vi "FOCUS_V42_H37.vi"(9 "X-pixels":sgl=256.0, 11 "Run":bool) -> (0 "Retrace pixels":sgl, 10 "Pixel Clock (Hz)":sgl)   [LabVIEW 2010] (continued)
            n1001 = Array Max & Min(array=w3025) -> (max value=w3029:dbl, min value=w3028:dbl)  [unwired: 2 out]
            n1002 = Greater?(x=w3029, y=w3022) -> (0:w3027:bool)
            n1003 = Less?(x=w3028, y=w3023) -> (x < y?=w3026:bool)
            n1004 = Or(x=w3027, y=w3026) -> (x .or. y?=w3024:bool)
            n1005 = case shown="False" w3024 {
              tunnel: [u32 16711680 u32 0] -> w3030
              frame True {
              }
              frame False {
                (unwired) u32 16756736
              }
            }
          }
        }
        n1006 = Bundle(w2040, w2041) -> (→"Galvos":cluster{dbl[], dbl[]})  [unwired: 1 in]
        n1007 = local read "frame/line indicator"() -> (w2025:u16)
        n1008 = local read "frame/line indicator"() -> (w1885:u16)
        n1009 = property class="DAQmx Buffer"(reference=w1952, error in=w1950, "Input:Buffer Size"=u32 10000000 ("Input.BufSize")) -> (reference out=w1951:refnum<k21>, error out=w1949:errorcluster)
        n1010 = Concatenate Strings(w1897, tag "/PXI_Trig2" ("source terminal")) -> (w1989:string)
        n1011 = call-poly <vilib>:"DAQmx Create Channel (CO-Pulse Generation-Ticks).vi"("high ticks"=w1877, "low ticks"=w1875, "counter"=w1935, "source of ticks"=w1929, "error in"=w1924, "initial delay"=w1878) -> ("task out"=w1961:refnum<k21>, "error out"=w1960:errorcluster)  [unwired: 8 in]
        n1012 = Greater Or Equal?(x=w2025, y=3.0) -> (x >= y?=w2024:bool)
        n1013 = Concatenate Strings(w1897, tag "/PXI_Trig2" ("destination terminal")) -> (w1993:string)
        n1014 = Bundle("Trigger?"="Trigger?", "Type"="Type", "Level [V]"="Level [V]", "slope"="slope") -> (w1908:T17)  [unwired: 1 in]
        n1015 = Type Cast(type=tag "" ("destination terminal"), x=w1989) -> (*(type *) &x=w1986:tag)
        n1016 = Concatenate Strings(w1897, tag "/10MHzRefClock" ("source terminal")) -> (w1998:string)
        n1017 = Type Cast(type=tag "" ("destination terminal"), x=w1993) -> (*(type *) &x=w1990:tag)
        n1018 = Type Cast(type=tag "" ("destination terminal"), x=w1998) -> (*(type *) &x=w1995:tag)
        n1019 = call-poly <vilib>:"DAQmx Timing (Implicit).vi"("task/channels in"=w1961, "sample mode"=w1959, "error in"=w1960) -> ("task out"=w1958:refnum<k21>, "error out"=w1957:errorcluster)  [unwired: 11 in]
        n1020 = case shown="3" w1885 {
          tunnel: [_ _ w3015 w3018 w3019] -> w2030
          frame 0, Default {
          }
          frame 1 {
          }
          frame 2 {
            n1021 = local read "Y-lines"() -> (w3016:sgl)
            n1022 = local read "Number of frames"() -> (w3017:sgl)
            n1023 = Multiply(x=w3016, y=w3017) -> (x*y=w3015:sgl)
          }
          frame 3 {
            n1024 = local read "Y-lines FreeLine"() -> (w3018:sgl)
          }
          frame 4 {
            n1025 = local read "Y-lines FreeLine"() -> (w3019:sgl)
          }
        }
        n1026 = local read "Fiberscope\nMode"() -> (w1894:bool)
        n1027 = case shown="False" w1894 {
          tunnel: w2024 -> [w2081 _]
          tunnel: w1947 -> [w2080 _]
          tunnel: [w2079 w2084] -> w1916
          frame False {
            n1028 = case shown="False" w2081 {
              tunnel: [w2082 w2083] -> w2079
              tunnel: w2080 -> [_ _]
              frame False {
                n1029 = local read "Pixel Clock (Hz)"() -> (w2082:sgl)
              }
              frame True {
                n1030 = local read "Pixel Clock (Hz) FreeLine"() -> (w2083:sgl)
              }
            }
          }
          frame True {
            n1031 = local read "Pixel Clock (Hz) FScope"() -> (w2084:sgl)
          }
        }
        n1032 = case shown="True" w1917 {
          tunnel: [_ w2978] -> w2014
          tunnel: [_ w2977] -> w2013
          tunnel: w1916 -> [_ w2974]
          tunnel: w1922 -> [_ w2962]
          frame False {
          }
          frame True {
            w2981 = 10123 items=["Finite Samples"=10178, "Continuous Samples"=10123, "Hardware Timed Single Point"=12522] ("sample mode")
            w2982 = 10171 items=["Rising"=10280, "Falling"=10171] ("edge")
            n1033 = local read "AI Device"() -> (w2949:tag)
            n1034 = Concatenate Strings(w2949, tag "/ai0," ("physical channels"), w2949, tag "/ai1," ("physical channels"), w2949, tag "/ai2," ("physical channels"), w2949, tag "/ai3" ("physical channels")) -> (w2971:string)
            n1035 = Type Cast(type=tag "" ("physical channels"), x=w2971) -> (*(type *) &x=w2968:tag)
            n1036 = local read "AO/DIO Device"() -> (w2952:tag)
            n1037 = call-poly <vilib>:"DAQmx Create Channel (AI-Voltage-Basic).vi"("maximum value"=10.0, "physical channels"=w2968, "error in"=w2962) -> ("task out"=w2979:refnum<k21>, "error out"=w2980:errorcluster)  [unwired: 11 in]
            n1038 = Concatenate Strings(tag "/" ("destination terminal"), w2952, tag "/ao/SampleClock" ("source")) -> (w2953:string)
            n1039 = Type Cast(type=tag "" ("source"), x=w2953) -> (*(type *) &x=w2951:tag)
            n1040 = call-poly <vilib>:"DAQmx Timing (Sample Clock).vi"("task/channels in"=w2979, "sample mode"=w2981, "rate"=w2974, "source"=w2951, "error in"=w2980) -> ("task out"=w2961:refnum<k21>, "error out"=w2960:errorcluster)  [unwired: 9 in]
            n1041 = property class="DAQmx Buffer"(reference=w2961, error in=w2960, "Input:Buffer Size"=u32 5000000 ("Input.BufSize")) -> (reference out=w2958:refnum<k21>, error out=w2959:errorcluster)
            n1042 = Concatenate Strings(tag "/" ("destination terminal"), w2952, tag "/ao/StartTrigger" ("source")) -> (w2967:string)
            n1043 = Type Cast(type=tag "" ("source"), x=w2967) -> (*(type *) &x=w2965:tag)
            n1044 = call-poly <vilib>:"DAQmx Start Trigger (Digital Edge).vi"("task/channels in"=w2958, "source"=w2965, "edge"=w2982, "error in"=w2959) -> ("task out"=w2976:refnum<k21>, "error out"=w2975:errorcluster)  [unwired: 10 in]
            n1045 = call <vilib>:"DAQmx Start Task.vi"("task/channels in"=w2976, "error in"=w2975) -> ("task out"=w2978:refnum<k21>, "error out"=w2977:errorcluster)  [unwired: 12 in]
          }
        }
        n1046 = call "AOConfigwriteDAQmx.vi"("AO.UseOnlyOnBrdMem"=FALSE, "TriggerCluster"=w1908, "Trigger Source"=w1907, "Sampling"=w1915, "rate"=w1916, "data"=w1889, "error in"=w1922, "RegenMode"=w2027, "Output.OnbrdBufSize"=w1947, "physical channels"=w2015) -> ("error out"=w2009:errorcluster, "task out"=w2008:refnum<k21>)
        n1047 = call <vilib>:"DAQmx Connect Terminals.vi"("source terminal"=w1995, "destination terminal"=w1990, "error in"=w2009) -> ("error out"=w2028:errorcluster)  [unwired: 12 in]
        n1048 = Concatenate Strings(w1897, tag "/ao/StartTrigger" ("source terminal")) -> (w1900:string)
        n1049 = call <vilib>:"DAQmx Start Task.vi"("task/channels in"=w1958, "error in"=w1957) -> ("task out"=w1956:refnum<k21>, "error out"=w1923:errorcluster)  [unwired: 12 in]
        n1050 = call-poly <vilib>:"DAQmx Timing (Sample Clock).vi"("task/channels in"=w1951, "sample mode"=w2012, "rate"=w1916, "source"=w1964, "error in"=w1949) -> ("task out"=w2011:refnum<k21>, "error out"=w2010:errorcluster)  [unwired: 9 in]
        n1051 = Concatenate Strings(w1897, tag "/PFI2" ("destination terminal")) -> (w1985:string)
        n1052 = Type Cast(type=tag "" ("destination terminal"), x=w1900) -> (*(type *) &x=w1896:tag)
        n1053 = Concatenate Strings(w1897, tag "/PFI5" ("destination terminal")) -> (w1977:string)
        n1054 = Concatenate Strings(w1897, tag "/PFI7" ("destination terminal")) -> (w1906:string)
        n1055 = local read "frame/line indicator"() -> (w2038:u16)
        n1056 = Type Cast(type=tag "" ("destination terminal"), x=w1985) -> (*(type *) &x=w1982:tag)
        n1057 = call <vilib>:"DAQmx Connect Terminals.vi"("source terminal"=w1986, "destination terminal"=w1982, "error in"=w2028) -> ("error out"=w1903:errorcluster)  [unwired: 12 in]
        n1058 = property on="Galvos" class="XYGraph (strict)"("Plot Area:Colors:FG Color"=w2042, "Plot Area:Colors:BG Color"=w2042) -> ()  [unwired: 2 in, 2 out]
        n1059 = Concatenate Strings(w1897, tag "/ao/SampleClock" ("source terminal")) -> (w1981:string)
        n1060 = Type Cast(type=tag "" ("destination terminal"), x=w1977) -> (*(type *) &x=w1974:tag)
        n1061 = Type Cast(type=tag "" ("destination terminal"), x=w1906) -> (*(type *) &x=w1901:tag)
        n1062 = call <vilib>:"DAQmx Connect Terminals.vi"("source terminal"=w1896, "destination terminal"=w1901, "error in"=w1903) -> ("error out"=w1902:errorcluster)  [unwired: 12 in]
        n1063 = call <vilib>:"DAQmx Start Task.vi"("task/channels in"=w2011, "error in"=w2010) -> ("task out"=w2017:refnum<k21>, "error out"=w2016:errorcluster)  [unwired: 12 in]
        n1064 = for {
          N: w2030 -> [_]
          tunnel: [w3020] -> w2031 mode=indexing
          i -> [w3020]
        }
        n1065 = Type Cast(type=tag "" ("destination terminal"), x=w1981) -> (*(type *) &x=w1978:tag)
        n1066 = call <vilib>:"DAQmx Connect Terminals.vi"("source terminal"=w1978, "destination terminal"=w1974, "error in"=w1902) -> ()  [unwired: 12 in, 1 out]
      }
    }
    n1067 = local read "Image3Array"() -> (w171:u8[][])
    n1068 = local read "Image4Array"() -> (w187:u8[][])
    n1069 = local read "Image1Array"() -> (w176:u8[][])
    n1070 = local read "Image2Array"() -> (w186:u8[][])
    n1071 = flat-sequence {
      tunnel: w176 -> [_]
      frame #0 {
        n1072 = property on="Property Node" class="VI"() -> ("VI Path"=w330:path)  [unwired: 2 in, 2 out]
        n1073 = Initialize Array(u8 0 ("x 2")) -> (w315:u8[])  [unwired: 1 in]
        n1074 = Strip Path(path=w330) -> (stripped path=w306:path)  [unwired: 1 out]
        n1075 = local read "VISA Sutter MP-285"() -> (w321:refnum<visa-resource-name>)
        n1076 = local read "MaiTai setting Path"() -> (w317:path)
        n1077 = local read "VISA XPG-ADC"() -> (w319:refnum<visa-resource-name>)
        n1078 = Strip Path(path=w306) -> ()  [unwired: 2 out]
        n1079 = local read "AO/DIO Device"() -> (w334:tag)
        n1080 = local read "AI Device"() -> (w327:tag)
        n1081 = Build Path(base path=w306, name or relative path="FOCUS.cfg") -> (appended path=w310:path)
        n1082 = Path To String(path=w317) -> (string=w316:string)
        n1083 = Type Cast(type="" ("name or relative path"), x=w319) -> (*(type *) &x=w318:string)
        n1084 = Type Cast(type="" ("name or relative path"), x=w321) -> (*(type *) &x=w320:string)
        n1085 = Type Cast(type=w315, x=w327) -> (*(type *) &x=w301:u8[])
        n1086 = Type Cast(type=w315, x=w316) -> (*(type *) &x=w314:u8[])
        n1087 = Type Cast(type=w315, x=w318) -> (*(type *) &x=w324:u8[])
        n1088 = Type Cast(type=w315, x=w320) -> (*(type *) &x=w325:u8[])
        n1089 = Type Cast(type=w315, x=w334) -> (*(type *) &x=w305:u8[])
        n1090 = Array Size(array=w301) -> (size(s)=w302:i32)
        n1091 = Array Size(array=w314) -> (size(s)=w313:i32)
        n1092 = Array Size(array=w305) -> (size(s)=w304:i32)
        n1093 = To Unsigned Byte Integer(number=w302) -> (unsigned 8bit integer=w300:u8)
        n1094 = To Unsigned Byte Integer(number=w313) -> (unsigned 8bit integer=w312:u8)
        n1095 = call <vilib>:"Open_Create_Replace File.vi"("advisory dialog? (display:T)"=FALSE, "function (open:0)"=T8."create or replace", "file path"=w310) -> ("error out"=w308:errorcluster, "refnum"=w309:refnum<file>)  [unwired: 5 in, 2 out]
        n1096 = To Unsigned Byte Integer(number=w304) -> (unsigned 8bit integer=w303:u8)
        n1097 = Build Array (concatenate)(w303, w305, w300, w301, w325, w324, w312, w314) -> (w326:u8[])
        n1098 = Write to Binary File(file (use dialog)=w309, data=w326, error in=w308, 5:FALSE ("prepend array or string size? (T)")) -> (refnum out=w328:refnum<file>, error out=w329:errorcluster)  [unwired: 2 in, 1 out]
        n1099 = Close File(refnum=w328, error in=w329) -> (error out=w332:errorcluster)  [unwired: 1 out]
        n1100 = call <vilib>:"Simple Error Handler.vi"("error in (no error)"=w332) -> ()  [unwired: 4 in, 5 out]
      }
    }
    n1101 = Equal?(x=w182, y=u16 4) -> (x = y?=w180:bool)
    n1102 = local read "ScanLineFreeLine"() -> (w198:sgl[][])
    n1103 = Index Array(array=w198, index (row)=0 ("disabled index (col)")) -> (element=w197:sgl[])  [unwired: 1 in]
    n1104 = Index Array(array=w198, index (row)=1 ("disabled index (col)")) -> (element=w178:sgl[])  [unwired: 1 in]
    n1105 = case shown="False" w180 {
      tunnel: [w335 w339] -> w179
      tunnel: w178 -> [w336 _]
      frame False {
        n1106 = Array Size(array=w336) -> (size(s)=w337:i32)
        n1107 = Initialize Array(sgl 0.0 ("element"), w337) -> (w335:sgl[])
      }
      frame True {
        n1108 = local read "Zsin3D"() -> (w339:sgl[])
      }
    }
    n1109 = Greater Or Equal?(x=w182, y=u16 3) -> (x >= y?=w183:bool)
    n1110 = local write "Ready?"(FALSE ("Ready?")) -> ()
    n1111 = property on="Image 2" class="IntGraph (strict)"() -> ("Color Table"=w289:u32[])  [unwired: 2 in, 2 out]
    n1112 = Interleave 1D Arrays(w197, w178, w179) -> (w193:sgl[])
    n1113 = local read "Positions"() -> (w192:sgl[])
    n1114 = local read "Focus"() -> (w208:bool)
    n1115 = local write "OpenShutter"(FALSE ("OpenShutter")) -> ()
    n1116 = local read "Channel selector"() -> (w160:u8)
    n1117 = Array Size(array=w193) -> (size(s)=w194:i32)
    n1118 = local write "Run"(w208) -> ()
    n1119 = Build Array (concatenate)(w194, w193, w192) -> (w185:sgl[])
    n1120 = flat-sequence {
      tunnel: [w431] -> w296
      tunnel: [w430] -> w163
      tunnel: [w398] -> w292
      tunnel: [w399] -> w291
      tunnel: w289 -> [w409]
      tunnel: w259 -> [w426]
      tunnel: w288 -> [w425]
      tunnel: [w424] -> w287
      tunnel: [w423] -> w286
      tunnel: w283 -> [w422]
      tunnel: w282 -> [w421]
      tunnel: [w400] -> w277
      tunnel: [w401] -> w276
      tunnel: [w387] -> w264
      tunnel: [w404] -> w219
      tunnel: [w403] -> w218
      tunnel: [w402] -> w210
      tunnel: w207 -> [w381]
      tunnel: w171 -> [w380]
      tunnel: w187 -> [w379]
      tunnel: w176 -> [w378]
      tunnel: w186 -> [w377]
      tunnel: w185 -> [w376]
      tunnel: w183 -> [w375]
      tunnel: w168 -> [w363]
      tunnel: [w363] -> w167
      tunnel: [w357] -> w161
      tunnel: w160 -> [w356]
      frame #0 {
        w408 = FALSE ("data")
        w420 = i8 -1 ("element")
        n1121 = local read "Mode selector"() -> (w372:u16)
        n1122 = local read "frame/line indicator"() -> (w428:u16)
        n1123 = local read "ImageSelector"() -> (w417:bool)
        n1124 = Split Number(x=w409) -> (lo(x)=w411:u16[])  [unwired: 1 out]
        n1125 = Split Number(x=w411) -> (lo(x)=w410:u8[])  [unwired: 1 out]
        n1126 = Equal?(x=w428, y=4) -> (x = y?=w362:bool)
        n1127 = Equal?(x=w372, y=4) -> (x = y?=w359:bool)
        n1128 = Or(x=w362, y=w363) -> (x .or. y?=w361:bool)
        n1129 = property on="Intensity" class="Slide (strict)"("Scale.Range:Maximum"="IntensityScaleMax") -> ()  [unwired: 2 in, 2 out]
        n1130 = Not(x=w359) -> (.not. x?=w360:bool)
        n1131 = And(x=w360, y=w361) -> (x .and. y?=w358:bool)
        n1132 = case shown="False" w358 {
          tunnel: [w456 _] -> w396
          tunnel: [w455 _] -> w397
          tunnel: w359 -> [w454 _]
          frame False {
            n1133 = case shown="True" w454 {
              tunnel: [w466 w479] -> w456
              tunnel: [w465 w478] -> w455
              frame False {
                n1134 = local read "AO/DIO Device"() -> (w462:tag)
                n1135 = Concatenate Strings(w462, tag "/ao3" ("physical channels")) -> (w460:string)
                n1136 = Type Cast(type=tag "" ("physical channels"), x=w460) -> (*(type *) &x=w458:tag)
                n1137 = call-poly <vilib>:"DAQmx Create Channel (AO-Voltage-Basic).vi"("physical channels"=w458) -> ("task out"=w463:refnum<k21>, "error out"=w464:errorcluster)  [unwired: 13 in]
                n1138 = local read "Intensity"() -> (w457:sgl)
                n1139 = call-poly <vilib>:"DAQmx Write (Analog DBL 1Chan 1Samp).vi"("task/channels in"=w463, "data"=w457, "error in"=w464) -> ("task out"=w466:refnum<k21>, "error out"=w465:errorcluster)  [unwired: 10 in, 1 out]
              }
              frame True {
                n1140 = local read "AO/DIO Device"() -> (w467:tag)
                n1141 = Concatenate Strings(w467, tag "/ao2," ("physical channels"), w467, tag "/ao3" ("physical channels")) -> (w474:string)
                n1142 = Type Cast(type=tag "" ("physical channels"), x=w474) -> (*(type *) &x=w472:tag)
                n1143 = call-poly <vilib>:"DAQmx Create Channel (AO-Voltage-Basic).vi"("physical channels"=w472) -> ("task out"=w476:refnum<k21>, "error out"=w477:errorcluster)  [unwired: 13 in]
                n1144 = local read "Intensity"() -> (w470:sgl)
                n1145 = Build Array(sgl 0.0 ("element"), w470) -> (w469:sgl[])
                n1146 = call-poly <vilib>:"DAQmx Write (Analog 1D DBL NChan 1Samp).vi"("task/channels in"=w476, "data"=w469, "error in"=w477) -> ("task out"=w479:refnum<k21>, "error out"=w478:errorcluster)  [unwired: 10 in, 1 out]
              }
            }
          }
          frame True {
          }
        }
        n1147 = local read "Fiberscope\nMode"() -> (w402:bool)
        n1148 = call "VISA MP-285 GetSet Speed.vi"("Input: Duty Cluster"=w381, "Input: Speed in microns/sec"="Sutter Speed [um/s]") -> ("Output: Duty Cluster"=w391:T18)  [unwired: 1 out]
        n1149 = call "VISA MP-285 Get Position.vi"("Input: Duty Cluster"=w391) -> ("Output: X axis (microns)"=w383:dbl, "Output: Y axis (microns)"=w384:dbl, "Output: Z axis (microns)"=w389:dbl, "Output: Duty Cluster"=w388:T18)
        n1150 = Multiply(x=w383, y="Sutter scale x") -> (x*y=→"x-positionstart (um)":dbl)
        n1151 = Multiply(x=w384, y="Sutter scale y") -> (x*y=→"y-positionstart (um)":dbl)
        n1152 = local read "frame scan finished?"() -> (w371:bool)
        n1153 = Multiply(x="Sutter scale z", y=w389) -> (x*y=w382:dbl)
        "z-positionstart (um)" <- w382
        n1154 = local read "AO/DIO Device"() -> (w414:tag)
        n1155 = property on="ImageSlide" class="Slide (strict)"() -> ("Scale.Range:Maximum"=w419:dbl, "Visible"=w418:bool)  [unwired: 2 in, 2 out]
        n1156 = case shown="True" w402 {
          tunnel: [_ w448] -> w404
          tunnel: [_ w447] -> w403
          frame False {
          }
          frame True {
            w442 = TRUE ("element")
            n1157 = local read "AO/DIO Device"() -> (w444:tag)
            n1158 = Concatenate Strings(w444, tag "/port2/line6," ("lines"), w444, tag "/port2/line7" ("lines")) -> (w453:string)
            n1159 = Type Cast(type=tag "" ("lines"), x=w453) -> (*(type *) &x=w451:tag)
            n1160 = call-poly <vilib>:"DAQmx Create Channel (DO-Digital Output).vi"("lines"=w451) -> ("task out"=w450:refnum<k21>, "error out"=w449:errorcluster)  [unwired: 13 in]
            n1161 = Build Array(w442, w442) -> (w443:bool[])
            n1162 = call-poly <vilib>:"DAQmx Write (Digital 1D Bool 1Chan 1Samp).vi"("task/channels in"=w450, "data"=w443, "error in"=w449) -> ("task out"=w448:refnum<k21>, "error out"=w447:errorcluster)  [unwired: 10 in, 1 out]
          }
        }
        n1163 = Concatenate Strings(w414, tag "/port1/line1" ("lines")) -> (w416:string)
        n1164 = local read "GetFirst"() -> (w385:bool)
        n1165 = local read "GetLast"() -> (w386:bool)
        n1166 = Type Cast(type=tag "" ("lines"), x=w416) -> (*(type *) &x=w412:tag)
        n1167 = And(x=w371, y="Go back?") -> (x .and. y?=w369:bool)
        n1168 = And(x=w385, y=w386) -> (x .and. y?=w374:bool)
        n1169 = call-poly <vilib>:"DAQmx Create Channel (DO-Digital Output).vi"("lines"=w412) -> ("task out"=w407:refnum<k21>, "error out"=w406:errorcluster)  [unwired: 13 in]
        "Shutter" <- w407
        n1170 = Or(x=w369, y=w374) -> (x .or. y?=w367:bool)
        n1171 = case shown="True" w367 {
          tunnel: w388 -> [w433 w441]
          tunnel: [w433 w440] -> w387
          tunnel: w382 -> [_ w438]
          tunnel: [FALSE ("IntDevUsed 2") FALSE ("IntDevUsed 2")] -> w368
          frame False {
          }
          frame True {
            n1172 = local read "FirstPosition"() -> (w437:sgl)
            n1173 = local read "Sutter scale z"() -> (w434:sgl)
            n1174 = Subtract(x=w437, y=w438) -> (x-y=w436:dbl)
            n1175 = Divide(x=w436, y=w434) -> (x/y=w439:dbl)
            n1176 = call "VISA MP-285 Step.vi"("Input: Duty Cluster"=w441, "Input: Delta Z axis (microns)"=w439) -> ("Output: Duty Cluster"=w440:T18)  [unwired: 2 in, 3 out]
          }
        }
        n1177 = local write "frame scan finished?"(w368) -> ()
        n1178 = local write "Shutter open"(w408) -> ()
        n1179 = call-poly <vilib>:"DAQmx Write (Digital Bool 1Line 1Point).vi"("task/channels in"=w407, "data"=w408, "error in"=w406) -> ("task out"=w394:refnum<k21>, "error out"=w395:errorcluster)  [unwired: 10 in, 1 out]
        n1180 = while {
          tunnel: ["Run"] -> w431
          tunnel: ["End experiment"] -> w430
          shift-right: [w581] -> _
          shift-left: w409 -> [w584]
          shift-right: [w579] -> _
          shift-left: FALSE ("Visible") -> [w580]
          tunnel: w426 -> [w578]
          tunnel: w425 -> [w577]
          tunnel: [w578] -> w424
          tunnel: [w577] -> w423
          tunnel: w422 -> [w575]
          tunnel: w421 -> [w567]
          shift-right: [w540] -> _
          shift-left: w420 -> [w541]
          shift-right: [w538] -> _
          shift-left: w420 -> [w539]
          tunnel: w419 -> [w537]
          tunnel: w418 -> [w536]
          shift-right: [w529] -> _
          shift-left: w417 -> [w528]
          shift-right: [w522] -> _
          shift-left: w410 -> [w523]
          tunnel: [w502] -> w401
          tunnel: [w501] -> w400
          tunnel: [w506] -> w399
          tunnel: [w505] -> w398
          tunnel: w397 -> [w508]
          tunnel: w396 -> [w507]
          tunnel: w395 -> [w504]
          tunnel: w394 -> [w503]
          tunnel: w380 -> [w488]
          tunnel: w379 -> [w487]
          tunnel: w378 -> [w489]
          tunnel: w377 -> [w490]
          tunnel: w376 -> [w493]
          tunnel: w375 -> [w491]
          tunnel: [w481] -> w357
          shift-right: [w480] -> _
          shift-left: w356 -> [w482]
          i -> [w527]
          stop <- w518 stop-if-true
          n1181 = local read "index (row)1"() -> (w546:i32)
          n1182 = property on="Image 2" class="IntGraph (strict)"() -> ("Color Table"=w583:u32[])  [unwired: 2 in, 2 out]
          n1183 = event shown="[0] Timeout" {
            selector: _ -> [_ _ _ _ _ _ _ _ _ _ _ _ _ _ _ _ _ _ _ _ _ _ _ _ _ _ _ _ _ _ _ _ _ _ _]
            dyn-events: _ -> [_ _ _ _ _ _ _ _ _ _ _ _ _ _ _ _ _ _ _ _ _ _ _ _ _ _ _ _ _ _ _ _ _ _ _]
            timeout: 0 -> [_ _ _ _ _ _ _ _ _ _ _ _ _ _ _ _ _ _ _ _ _ _ _ _ _ _ _ _ _ _ _ _ _ _ _]
            tunnel: [FALSE ("Fiberscope\nMode") TRUE ("Fiberscope\nMode") TRUE ("Fiberscope\nMode") TRUE ("Fiberscope\nMode") TRUE ("Fiberscope\nMode") TRUE ("Fiberscope\nMode") TRUE ("Fiberscope\nMode") TRUE ("Fiberscope\nMode") TRUE ("Fiberscope\nMode") TRUE ("Fiberscope\nMode") TRUE ("Fiberscope\nMode") TRUE ("Fiberscope\nMode") TRUE ("Fiberscope\nMode") TRUE ("Fiberscope\nMode") TRUE ("Fiberscope\nMode") TRUE ("Fiberscope\nMode") TRUE ("Fiberscope\nMode") TRUE ("Fiberscope\nMode") TRUE ("Fiberscope\nMode") TRUE ("Fiberscope\nMode") TRUE ("Fiberscope\nMode") TRUE ("Fiberscope\nMode") TRUE ("Fiberscope\nMode") TRUE ("Fiberscope\nMode") TRUE ("Fiberscope\nMode") TRUE ("Fiberscope\nMode") TRUE ("Fiberscope\nMode") TRUE ("Fiberscope\nMode") TRUE ("Fiberscope\nMode") FALSE ("Fiberscope\nMode") _ FALSE ("Fiberscope\nMode") FALSE ("Fiberscope\nMode") FALSE ("Fiberscope\nMode") FALSE ("Fiberscope\nMode")] -> w510
            tunnel: [_ _ _ _ _ _ _ _ w657 _ _ _ _ _ _ _ _ _ _ _ _ _ _ _ _ _ _ _ _ _ _ _ _ _ _] -> w509
            tunnel: w508 -> [w615 w620 w625 w630 w635 w640 w645 w650 w655 w661 w666 w671 w676 w681 w686 w691 w696 w701 w706 w711 w716 w721 w726 w731 w736 w741 w746 w751 w757 w765 w770 w777 w797 w802 w809]
            tunnel: w507 -> [w616 w621 w626 w631 w636 w641 w646 w651 w656 w662 w667 w672 w677 w682 w687 w692 w697 w702 w707 w712 w717 w722 w727 w732 w737 w742 w747 w752 w758 w764 w771 w778 w798 w803 w810]
            tunnel: [w615 w620 w625 w630 w635 w640 w645 w650 w655 w661 w666 w671 w676 w681 w686 w691 w696 w701 w706 w711 w716 w721 w726 w731 w736 w741 w746 w751 w757 w763 w770 w777 w797 w802 w809] -> w506
            tunnel: [w616 w621 w626 w631 w636 w641 w646 w651 w656 w662 w667 w672 w677 w682 w687 w692 w697 w702 w707 w712 w717 w722 w727 w732 w737 w742 w747 w752 w758 w762 w771 w778 w798 w803 w810] -> w505
            tunnel: w504 -> [w613 w618 w623 w628 w633 w638 w643 w648 w653 w659 w664 w669 w674 w679 w684 w689 w694 w699 w704 w709 w714 w719 w724 w729 w734 w739 w744 w749 w755 w760 w774 w775 w795 w800 w807]
            tunnel: w503 -> [w614 w619 w624 w629 w634 w639 w644 w649 w654 w660 w665 w670 w675 w680 w685 w690 w695 w700 w705 w710 w715 w720 w725 w730 w735 w740 w745 w750 w756 w761 w773 w776 w796 w801 w808]
            tunnel: [w613 w618 w623 w628 w633 w638 w643 w648 w653 w659 w664 w669 w674 w679 w684 w689 w694 w699 w704 w709 w714 w719 w724 w729 w734 w739 w744 w749 w755 w760 w769 w775 w795 w800 w807] -> w502
            tunnel: [w614 w619 w624 w629 w634 w639 w644 w649 w654 w660 w665 w670 w675 w680 w685 w690 w695 w700 w705 w710 w715 w720 w725 w730 w735 w740 w745 w750 w756 w761 w768 w776 w796 w801 w808] -> w501
            tunnel: w493 -> [_ _ _ _ _ _ _ _ _ _ _ _ _ _ _ _ _ _ _ _ _ _ _ _ _ _ _ _ _ _ _ _ w791 _ _]
            tunnel: w491 -> [_ _ _ _ _ _ _ _ _ _ _ _ _ _ _ _ _ _ _ _ _ _ _ _ _ _ _ _ _ _ _ _ w787 _ _]
            tunnel: w489 -> [_ _ _ _ _ _ _ _ _ _ _ _ _ _ _ _ _ _ _ _ _ _ _ _ _ _ _ _ _ _ _ _ _ _ _]
            tunnel: w490 -> [_ _ _ _ _ _ _ _ _ _ _ _ _ _ _ _ _ _ _ _ _ _ _ _ _ _ _ _ _ _ _ _ _ _ _]
            tunnel: w488 -> [_ _ _ _ _ _ _ _ _ _ _ _ _ _ _ _ _ _ _ _ _ _ _ _ _ _ _ _ _ _ _ _ _ _ _]
            tunnel: w487 -> [_ _ _ _ _ _ _ _ _ _ _ _ _ _ _ _ _ _ _ _ _ _ _ _ _ _ _ _ _ _ _ _ _ _ _]
            event Timeout {
              n1184 = event-data() -> ()  [unwired: 1 in, 2 out]
            }
            event "Mode selector": Value Change {
              n1185 = event-data() -> ()  [unwired: 1 in, 2 out]
            }
            event "Scan format": Value Change {
              n1186 = event-data() -> ()  [unwired: 1 in, 2 out]
            }
            event "Measurement cursor check box": Value Change {
              n1187 = event-data() -> ()  [unwired: 1 in, 2 out]
            }
            event "View line\ncheck box": Value Change {
              n1188 = event-data() -> ()  [unwired: 1 in, 2 out]
            }
            event "X-pixels": Value Change {
              n1189 = event-data() -> ()  [unwired: 1 in, 2 out]
            }
            event "Y-lines": Value Change {
              n1190 = event-data() -> ()  [unwired: 1 in, 2 out]
            }
            event "line scan time (ms)": Value Change {
              n1191 = event-data() -> ()  [unwired: 1 in, 2 out]
            }
            event "Type": Value Change {
              n1192 = event-data() -> ("NewVal"=w657:bool)  [unwired: 1 in, 1 out]
            }
            event "Level [V]": Value Change {
              n1193 = event-data() -> ()  [unwired: 1 in, 2 out]
            }
            event "Number of stacks": Value Change {
              n1194 = event-data() -> ()  [unwired: 1 in, 2 out]
            }
            event "new FreeLine?": Value Change {
              n1195 = event-data() -> ()  [unwired: 1 in, 2 out]
            }
            event "FocusModeSelector": Value Change {
              n1196 = event-data() -> ()  [unwired: 1 in, 2 out]
            }
            event "Trigger?": Value Change {
              n1197 = event-data() -> ()  [unwired: 1 in, 2 out]
            }
            event "Number of frames": Value Change {
              n1198 = event-data() -> ()  [unwired: 1 in, 2 out]
            }
            event "Averaging": Value Change {
              n1199 = event-data() -> ()  [unwired: 1 in, 2 out]
            }
            event "z-step (um)": Value Change {
              n1200 = event-data() -> ()  [unwired: 1 in, 2 out]
            }
            event "Fiberscope\nMode": Value Change {
              n1201 = event-data() -> ()  [unwired: 1 in, 3 out]
            }
            event "NewScanpattern": Value Change {
              n1202 = event-data() -> ()  [unwired: 1 in, 3 out]
            }
            event "Scan format FScope": Value Change {
              n1203 = event-data() -> ()  [unwired: 1 in, 3 out]
            }
            event "X dim": Value Change {
              n1204 = event-data() -> ()  [unwired: 1 in, 3 out]
            }
            event "Y dim": Value Change {
              n1205 = event-data() -> ()  [unwired: 1 in, 3 out]
            }
            event "Mode selectorFScope": Value Change {
              n1206 = event-data() -> ()  [unwired: 1 in, 3 out]
            }
            event "Number of Frames": Value Change {
              n1207 = event-data() -> ()  [unwired: 1 in, 3 out]
            }
            event "Averaging": Value Change {
              n1208 = event-data() -> ()  [unwired: 1 in, 3 out]
            }
            event "LS X/Y": Value Change {
              n1209 = event-data() -> ()  [unwired: 1 in, 3 out]
            }
            event "Number of Stacks": Value Change {
              n1210 = event-data() -> ()  [unwired: 1 in, 3 out]
            }
            event "Time interval [s]": Value Change {
              n1211 = event-data() -> ()  [unwired: 1 in, 3 out]
            }
            event "Scanpattern": Value Change {
              n1212 = event-data() -> ()  [unwired: 1 in, 3 out]
            }
            event "Intensity": Value Change {
              n1213 = event-data() -> ()  [unwired: 1 in, 2 out]
              n1214 = local read "Intensity"() -> (w759:sgl)
              n1215 = call-poly <vilib>:"DAQmx Write (Analog DBL 1Chan 1Samp).vi"("task/channels in"=w764, "data"=w759, "error in"=w765) -> ("task out"=w762:refnum<k21>, "error out"=w763:errorcluster)  [unwired: 10 in, 1 out]
              n1216 = Build Array(sgl 0.0 ("value"), w759) -> ()  [unwired: 1 out]
            }
            event "OpenShutter": Value Change {
              n1217 = event-data() -> ()  [unwired: 1 in, 2 out]
              n1218 = call-poly <vilib>:"DAQmx Write (Digital Bool 1Line 1Point).vi"("task/channels in"=w773, "data"="OpenShutter", "error in"=w774) -> ("task out"=w768:refnum<k21>, "error out"=w769:errorcluster)  [unwired: 10 in, 1 out]
              n1219 = local write "Shutter open"("OpenShutter") -> ()
            }
            event "2Ch\noverlay\nbutton": Mouse Down {
              n1220 = event-data() -> ()  [unwired: 1 in, 2 out]
              n1221 = call "OverlayFOCUS.vi"() -> ()  [unwired: 1 in]
            }
            event "Save? 2": Value Change {
              n1222 = event-data() -> ()  [unwired: 1 in, 1 out]
              n1223 = property on="Property Node" class="VI"() -> ("VI Path"=w784:path)  [unwired: 2 in, 2 out]
              n1224 = local read "FilePath"() -> (w789:path)
              n1225 = local read "NotebookFile"() -> (w781:path)
              n1226 = local read "Header"() -> (w785:u8[])
              n1227 = local read "BaseFilename"() -> (w790:string)
              n1228 = Bundle("BaseFilename"=w790, "FilePath"=w789, "Autoincrement Filename"="Autoincrement Filename", w787) -> (w786:T19)  [unwired: 1 in]
              n1229 = call "SavenewFOCUS.vi"("source path"=w784, "Header"=w785, "Positions"=w791, "Parameters"=w786) -> ("Data directory out"=w780:path, "name"=→"Filename":string, "basename out"=w793:string)
              n1230 = local write "BaseFilename"(w793) -> ()
              n1231 = local write "FilePath"(w780) -> ()
              n1232 = call "SaveNotebookFOCUS.vi"("Notebook Window"="Notebook Window", "NotebookFile"=w781, "FilePathCurrent"=w780) -> ("NotebookFile"=w783:path)
              n1233 = local write "NotebookFile"(w783) -> ()
              "Save?" <- TRUE ("Save?")
            }
            event "Different Integrator Setting": Mouse Down {
              n1234 = event-data() -> ()  [unwired: 1 in, 1 out]
              n1235 = call "IntegratorSetting.vi"("VISA resource name"="VISA XPG-ADC") -> ()
            }
            event "MaiTai setting": Mouse Down {
              n1236 = event-data() -> ()  [unwired: 1 in, 1 out]
              n1237 = call "RunAppl.vi"("Path"="MaiTai setting Path") -> ()
            }
          }
          n1238 = local read "Channel selector"() -> (w480:u8)
          n1239 = Subtract(x=w546, y="SlideHorizontal") -> (x-y=w545:u32)
          n1240 = case shown="False" "Different colour table" {
            tunnel: [w1416 w1433] -> w515
            tunnel: "Default colour table" -> [w1417 _]
            tunnel: w584 -> [w1415 w1435]
            tunnel: "reset?" -> [_ w1441]
            tunnel: w583 -> [w1414 _]
            tunnel: [w1413 w1434] -> w581
            tunnel: w580 -> [w1412 w1439]
            tunnel: [w1411 w1438] -> w579
            tunnel: [w1409 w1432] -> w522
            tunnel: w523 -> [w1410 w1429]
            tunnel: [w1407 w1428] -> w484
            tunnel: [w1408 w1427] -> w485
            frame False {
              n1241 = case shown="True" w1417 {
                tunnel: [w1421 w1422] -> w1416
                tunnel: w1415 -> [w1420 _]
                tunnel: w1414 -> [w1421 _]
                tunnel: [w1420 w1422] -> w1413
                tunnel: w1412 -> [w1419 w1424]
                tunnel: [w1419 w1424] -> w1411
                tunnel: w1410 -> [w1418 _]
                tunnel: [w1418 u8[] [255, 0, 1, 2, 3, 4, 5, 6, 7, 8, 9, 10, 11, 12, 13, 14, 15, 16, 17, 18, 19, 20, 21, 22, 23, 24, 25, 26, 27, 28, 29, 30, 31, 32, 33, 34, 35, 36, 37, 38, 39, 40, 41, 42, 43, 44, 45, 46, 47, 48, 49, 50, 51, 52, 53, 54, 55, 56, 57, 58, 59, 60, 61, 62, 64, 65, 66, 67, 68, 69, 70, 71, 72, 73, 74, 75, 76, 77, 78, 79, 80, 81, 82, 83, 84, 85, 86, 87, 88, 89, 90, 91, 92, 93, 94, 95, 96, 97, 98, 99, 100, 101, 102, 103, 104, 105, 106, 107, 108, 109, 110, 111, 112, 113, 114, 115, 116, 117, 118, 119, 120, 121, 122, 123, 124, 125, 126, 127, 128, 129, 130, 131, 132, 133, 134, 135, 136, 137, 138, 139, 140, 141, 142, 143, 144, 145, 146, 147, 148, 149, 150, 151, 152, 153, 154, 155, 156, 157, 158, 159, 160, 161, 162, 163, 164, 165, 166, 167, 168, 169, 170, 171, 172, 173, 174, 175, 176, 177, 178, 179, 180, 181, 182, 183, 184, 185, 186, 187, 188, 189, 191, 192, 193, 194, 195, 196, 197, 198, 199, 200, 201, 202, 203, 204, 205, 206, 207, 208, 209, 210, 211, 212, 213, 214, 215, 216, 217, 218, 219, 220, 221, 222, 223, 224, 225, 226, 227, 228, 229, 230, 231, 232, 233, 234, 235, 236, 237, 238, 239, 240, 241, 242, 243, 244, 245, 246, 247, 248, 249, 250, 251, 252, 253, 254, 255, 0] ("ColorFactor")] -> w1409
                frame False {
                }
                frame True {
                  w1422 = u32[] [255, 0, 65793, 131586, 197379, 263172, 328965, 394758, 460551, 526344, 592137, 657930, 723723, 789516, 855309, 921102, 986895, 1052688, 1118481, 1184274, 1250067, 1315860, 1381653, 1447446, 1513239, 1579032, 1644825, 1710618, 1776411, 1842204, 1907997, 1973790, 2039583, 2105376, 2171169, 2236962, 2302755, 2368548, 2434341, 2500134, 2565927, 2631720, 2697513, 2763306, 2829099, 2894892, 2960685, 3026478, 3092271, 3158064, 3223857, 3289650, 3355443, 3421236, 3487029, 3552822, 3618615, 3684408, 3750201, 3815994, 3881787, 3947580, 4013373, 4079166, 4210752, 4276545, 4342338, 4408131, 4473924, 4539717, 4605510, 4671303, 4737096, 4802889, 4868682, 4934475, 5000268, 5066061, 5131854, 5197647, 5263440, 5329233, 5395026, 5460819, 5526612, 5592405, 5658198, 5723991, 5789784, 5855577, 5921370, 5987163, 6052956, 6118749, 6184542, 6250335, 6316128, 6381921, 6447714, 6513507, 6579300, 6645093, 6710886, 6776679, 6842472, 6908265, 6974058, 7039851, 7105644, 7171437, 7237230, 7303023, 7368816, 7434609, 7500402, 7566195, 7631988, 7697781, 7763574, 7829367, 7895160, 7960953, 8026746, 8092539, 8158332, 8224125, 8289918, 8355711, 8421504, 8487297, 8553090, 8618883, 8684676, 8750469, 8816262, 8882055, 8947848, 9013641, 9079434, 9145227, 9211020, 9276813, 9342606, 9408399, 9474192, 9539985, 9605778, 9671571, 9737364, 9803157, 9868950, 9934743, 10000536, 10066329, 10132122, 10197915, 10263708, 10329501, 10395294, 10461087, 10526880, 10592673, 10658466, 10724259, 10790052, 10855845, 10921638, 10987431, 11053224, 11119017, 11184810, 11250603, 11316396, 11382189, 11447982, 11513775, 11579568, 11645361, 11711154, 11776947, 11842740, 11908533, 11974326, 12040119, 12105912, 12171705, 12237498, 12303291, 12369084, 12434877, 12566463, 12632256, 12698049, 12763842, 12829635, 12895428, 12961221, 13027014, 13092807, 13158600, 13224393, 13290186, 13355979, 13421772, 13487565, 13553358, 13619151, 13684944, 13750737, 13816530, 13882323, 13948116, 14013909, 14079702, 14145495, 14211288, 14277081, 14342874, 14408667, 14474460, 14540253, 14606046, 14671839, 14737632, 14803425, 14869218, 14935011, 15000804, 15066597, 15132390, 15198183, 15263976, 15329769, 15395562, 15461355, 15527148, 15592941, 15658734, 15724527, 15790320, 15856113, 15921906, 15987699, 16053492, 16119285, 16185078, 16250871, 16316664, 16382457, 16448250, 16514043, 16579836, 16645629, 16711422, 16777215, 16711680] ("Array")
                  n1242 = local write "Default colour table"(FALSE ("Visible")) -> ()
                  n1243 = local write "reset?"(125.0 ("element")) -> ()
                  n1244 = property on="Image 2" class="IntGraph (strict)"("Color Table"=w1422) -> ()  [unwired: 2 in, 2 out]
                  n1245 = property on="Image 1" class="IntGraph (strict)"("Color Table"=w1422) -> ()  [unwired: 2 in, 2 out]
                }
              }
              n1246 = local read "CT1"() -> (w1408:bool)
              n1247 = local read "CT2"() -> (w1407:bool)
            }
            frame True {
              n1248 = local read "Image 1"() -> (w1431:u8[][])
              n1249 = local read "Image 2"() -> (w1430:u8[][])
              n1250 = call "ColorTableGeneratorBWCLFOCUS.vi"("ColourFactor"=w1429, "Image 2"=w1430, "Stop?"=w1439, "Reset"=w1441, "old colour table"=w1435, "Image 1"=w1431) -> ("ColourFactor"=w1432:u32[], "New ClTb"=w1437:bool, 2:w1436:u32[], "Stop?"=w1438:bool, "Ch2"=w1428:bool, "Ch1"=w1427:bool)
              n1251 = local write "Different colour table"(w1438) -> ()
              n1252 = local write "reset?"(0.0 ("element")) -> ()
              n1253 = case shown="True" w1437 {
                tunnel: w1436 -> [w1443 w1444]
                tunnel: [w1443 w1444] -> w1433
                tunnel: [w1442 w1444] -> w1434
                tunnel: w1435 -> [w1442 _]
                frame False {
                }
                frame True {
                }
              }
            }
          }
          "CT2" <- w484
          "CT1" <- w485
          n1254 = local read "Average1"() -> (w557:i32)
          n1255 = property on="Image 3" class="IntGraph (strict)"("Active Cursor"=u32 0, "Cursor.Visible"=TRUE, "Cursor.Cursor Color"=u32 16711680, "Cursor.Cursor Position:Cursor X"=w545, "Cursor.Cursor Position:Cursor Y"=i8 -1 ("Active Cursor")) -> ()  [unwired: 2 in, 2 out]
          n1256 = Not Equal?(x=w482, y=w480) -> (x != y?=w481:bool)
          n1257 = Add(x=w545, y=w557) -> (x+y=w566:u32)
          n1258 = property on="Image 3" class="IntGraph (strict)"("Active Cursor"=u32 1, "Cursor.Visible"=TRUE, "Cursor.Cursor Color"=u32 16711680, "Cursor.Cursor Position:Cursor X"=w566, "Cursor.Cursor Position:Cursor Y"=i8 -1 ("Active Cursor")) -> ()  [unwired: 2 in, 2 out]
          n1259 = property on="Level [V]" class="DigNum (strict)"("Visible"=w509) -> ()  [unwired: 2 in, 2 out]
          n1260 = local read "index (row)2"() -> (w543:i32)
          n1261 = local read "frame/line indicator"() -> (w525:u16)
          n1262 = local read "Overlay Images"() -> (w576:bool)
          n1263 = Compound Arithmetic op=OR("Run", w510, "Open?", "End experiment", "Focus", w481) -> (w518:bool)
          n1264 = case shown="True" "Focus" {
            frame False {
            }
            frame True {
              w812 = u16 0 items=["Focus mode", "Frame scan", "Straight line scan", "FreeLine 2D", "Frame scan piezo", "FreeLine 3D"] ("Mode selector")
              n1265 = local write "Mode selector"(w812) -> ()
            }
          }
          n1266 = Subtract(x=w543, y="SlideHorizontal") -> (x-y=w542:u32)
          n1267 = Not Or(1:w484, 2:w485) -> (0:w483:bool)
          n1268 = Equal?(x=w525, y=u16 3) -> (x = y?=w533:bool)
          n1269 = And(x=w485, y=w484) -> (x .and. y?=w486:bool)
          n1270 = local read "Average2"() -> (w556:i32)
          n1271 = case shown="False" w483 {
            tunnel: w576 -> [w591 _]
            tunnel: w522 -> [w590 _]
            tunnel: w515 -> [w589 _]
            tunnel: w486 -> [w588 _]
            tunnel: w485 -> [w587 _]
            frame False {
              n1272 = case shown="False" w591 {
                tunnel: w589 -> [w595 _]
                tunnel: w590 -> [_ w604]
                tunnel: w588 -> [w594 _]
                tunnel: w587 -> [w593 _]
                frame False {
                  w592 = FALSE ("CT1")
                  n1273 = case shown="False" w594 {
                    tunnel: w595 -> [w597 w599]
                    tunnel: w593 -> [_ w598]
                    frame True {
                      n1274 = property on="Image 2" class="IntGraph (strict)"("Color Table"=w597) -> ()  [unwired: 2 in, 2 out]
                      n1275 = property on="Image 1" class="IntGraph (strict)"("Color Table"=w597) -> ()  [unwired: 2 in, 2 out]
                      "colour table" <- w597
                    }
                    frame False {
                      n1276 = case shown="False" w598 {
                        tunnel: w599 -> [w600 w601]
                        frame False {
                          n1277 = property on="Image 2" class="IntGraph (strict)"("Color Table"=w600) -> ()  [unwired: 2 in, 2 out]
                          "colour table 2" <- w600
                        }
                        frame True {
                          n1278 = local write "colour table"(w601) -> ()
                          n1279 = property on="Image 1" class="IntGraph (strict)"("Color Table"=w601) -> ()  [unwired: 2 in, 2 out]
                        }
                      }
                    }
                  }
                  n1280 = local write "CT1"(w592) -> ()
                  n1281 = local write "CT2"(w592) -> ()
                  n1282 = property on="Image 2" class="IntGraph (strict)"("Visible"=TRUE) -> ()  [unwired: 2 in, 2 out]
                }
                frame True {
                  n1283 = call "ColourFactor.vi"("ColorFactor"=w604, "ColorTable"=u32[] [255, 327680, 328192, 328960, 132352, 1280, 655360, 656640, 657920, 330240, 2560, 983040, 985088, 986880, 528128, 3840, 1310720, 1313280, 1315840, 660480, 5120, 1638400, 1641472, 1644800, 792832, 6400, 1966080, 1969920, 1973760, 990720, 7680, 2293760, 2298368, 2302720, 1188608, 8960, 2621440, 2626560, 2631680, 1320960, 10240, 2949120, 2954752, 2960640, 1453312, 11520, 3276800, 3283200, 3289600, 1651200, 12800, 3604480, 3611648, 3618560, 1849088, 14080, 3932160, 3939840, 3947520, 1981440, 15360, 4259840, 4268032, 4276480, 2113792, 16640, 4587520, 4596480, 4605440, 2311680, 17920, 4915200, 4924928, 4934400, 2509568, 19200, 5242880, 5253120, 5263360, 2641920, 20480, 5570560, 5581312, 5592320, 2774272, 21760, 5898240, 5909760, 5921280, 2972160, 23040, 6225920, 6238208, 6250240, 3170048, 24320, 6553600, 6566400, 6579200, 3302400, 25600, 6881280, 6894592, 6908160, 3434752, 26880, 7208960, 7223040, 7237120, 3632640, 28160, 7536640, 7551488, 7566080, 3830528, 29440, 7864320, 7879680, 7895040, 3962880, 30720, 8192000, 8207872, 8224000, 4095232, 32000, 8519680, 8536320, 8552960, 4293120, 33280, 8847360, 8864768, 8881920, 4491008, 34560, 9175040, 9192960, 9210880, 4623360, 35840, 9502720, 9521152, 9539840, 4755712, 37120, 9830400, 9849600, 9868800, 4953600, 38400, 10158080, 10178048, 10197760, 5151488, 39680, 10485760, 10506240, 10526720, 5283840, 40960, 10813440, 10834432, 10855680, 5416192, 42240, 11141120, 11162880, 11184640, 5614080, 43520, 11468800, 11491328, 11513600, 5811968, 44800, 11796480, 11819520, 11842560, 5944320, 46080, 12124160, 12147712, 12171520, 6076672, 47360, 12451840, 12476160, 12500480, 6274560, 48640, 12779520, 12804608, 12829440, 6472448, 49920, 13107200, 13132800, 13158400, 6604800, 51200, 13434880, 13460992, 13487360, 6737152, 52480, 13762560, 13789440, 13816320, 6935040, 53760, 14090240, 14117888, 14145280, 7132928, 55040, 14417920, 14446080, 14474240, 7265280, 56320, 14745600, 14774272, 14803200, 7397632, 57600, 15073280, 15102720, 15132160, 7595520, 58880, 15400960, 15431168, 15461120, 7793408, 60160, 15728640, 15759360, 15790080, 7925760, 61440, 16056320, 16087552, 16119040, 8058112, 62720, 16384000, 16416000, 16448000, 8256000, 64000, 16763080, 16768200, 16777215, 14483400, 13172680] ("Array")) -> ("ColorTable"=w603:u32[])
                  n1284 = local write "colour table"(w603) -> ()
                  n1285 = property on="Image 2" class="IntGraph (strict)"("Visible"=FALSE) -> ()  [unwired: 2 in, 2 out]
                  n1286 = property on="Image 1" class="IntGraph (strict)"("Color Table"=w603) -> ()  [unwired: 2 in, 2 out]
                }
              }
            }
            frame True {
            }
          }
          n1287 = Equal?(x=w525, y=u16 4) -> (x = y?=w524:bool)
          n1288 = case shown="False" "ImageSelector" {
            selector: "ImageSelector" -> [w831 w842]
            tunnel: w537 -> [_ w840]
            tunnel: w536 -> [_ w841]
            tunnel: [w829 w841] -> w535
            tunnel: [w828 w840] -> w531
            tunnel: w533 -> [w827 _]
            tunnel: w524 -> [w826 _]
            frame False {
              n1289 = property on="Image 3" class="IntGraph (strict)"("Visible"=w831) -> ()  [unwired: 2 in, 2 out]
              n1290 = property on="Histogram1" class="XYGraph (strict)"("Visible"=w831) -> ()  [unwired: 2 in, 2 out]
              n1291 = property on="Image 4" class="IntGraph (strict)"("Visible"=w831) -> ()  [unwired: 2 in, 2 out]
              n1292 = property on="Histogram2" class="XYGraph (strict)"("Visible"=w831) -> ()  [unwired: 2 in, 2 out]
              n1293 = case shown="False" w827 {
                tunnel: [w833 sgl 0.0] -> w828
                tunnel: w826 -> [w832 _]
                frame False {
                  n1294 = case shown="False" w832 {
                    tunnel: [w834 w835] -> w833
                    frame False {
                      n1295 = local read "ImageSlideMax"() -> (w834:sgl)
                    }
                    frame True {
                      n1296 = local read "Number of frames"() -> (w836:sgl)
                      n1297 = Decrement(x=w836) -> (x-1=w835:sgl)
                    }
                  }
                }
                frame True {
                }
              }
              n1298 = Less Or Equal To 0?(x=w828) -> (x <= 0?=w830:bool)
              n1299 = case shown="False" w830 {
                tunnel: [TRUE ("Visible") FALSE ("Visible")] -> w829
                frame False {
                }
                frame True {
                }
              }
            }
            frame True {
              n1300 = property on="Image 3" class="IntGraph (strict)"("Visible"=w842) -> ()  [unwired: 2 in, 2 out]
              n1301 = property on="Histogram1" class="XYGraph (strict)"("Visible"=w842) -> ()  [unwired: 2 in, 2 out]
              n1302 = property on="Image 4" class="IntGraph (strict)"("Visible"=w842) -> ()  [unwired: 2 in, 2 out]
              n1303 = property on="Histogram2" class="XYGraph (strict)"("Visible"=w842) -> ()  [unwired: 2 in, 2 out]
            }
          }
          n1304 = case shown="False" "XScale" {
            tunnel: [w820 w825] -> w569
            tunnel: [w822 0.0 ("Scale.Range:Minimum")] -> w571
            tunnel: [TRUE ("Ready?") FALSE ("Ready?")] -> w570
            frame False {
              n1305 = local read "X-pixels FreeLine"() -> (w821:sgl)
              n1306 = local read "Y-lines FreeLine"() -> (w820:sgl)
              n1307 = Subtract(x=w821, y=w820) -> (x-y=w822:sgl)
            }
            frame True {
              n1308 = local read "X-pixels FreeLine"() -> (w825:sgl)
            }
          }
          n1309 = property on="Image 4" class="IntGraph (strict)"("Active Cursor"=u32 0, "Cursor.Visible"=TRUE, "Cursor.Cursor Color"=u32 16711680, "Cursor.Cursor Position:Cursor X"=w542, "Cursor.Cursor Position:Cursor Y"=i8 -1 ("Active Cursor")) -> ()  [unwired: 2 in, 2 out]
          n1310 = Add(x=w542, y=w556) -> (x+y=w547:u32)
          n1311 = Not Equal?(x=w528, y="ImageSelector") -> (x != y?=w520:bool)
          n1312 = property on="Image 4" class="IntGraph (strict)"("Active Cursor"=u32 1, "Cursor.Visible"=TRUE, "Cursor.Cursor Color"=u32 16711680, "Cursor.Cursor Position:Cursor X"=w547, "Cursor.Cursor Position:Cursor Y"=i8 -1 ("Active Cursor")) -> ()  [unwired: 2 in, 2 out]
          n1313 = property on="Image 3" class="IntGraph (strict)"("X Scale.Range:Maximum"=w569) -> ()  [unwired: 2 in, 2 out]
          n1314 = local read "Mode selector"() -> (w498:u16)
          n1315 = property on="SlideHorizontal" class="Slide (strict)"("Scale.Range:Minimum"=0.0, "Scale.Range:Maximum"=w571) -> ()  [unwired: 2 in, 2 out]
          n1316 = Equal To 0?(x=w527) -> (x = 0?=w492:bool)
          n1317 = Or(x=w492, y=w520) -> ()  [unwired: 1 out]
          n1318 = property on="Image 4" class="IntGraph (strict)"("X Scale.Range:Maximum"=w569) -> ()  [unwired: 2 in, 2 out]
          n1319 = Equal?(x=u16 2, y=w498) -> (x = y?=w495:bool)
          n1320 = And(x=w495, y="Y-Scale") -> (x .and. y?=w494:bool)
          n1321 = case shown="True" w494 {
            tunnel: [w607 w610] -> w500
            tunnel: ["ImageSlide" u32 0 ("ImageSlide")] -> w499
            frame False {
              n1322 = local read "X-pixels"() -> (w608:sgl)
              n1323 = Decrement(x=w608) -> (x-1=w607:sgl)
            }
            frame True {
              n1324 = local read "Number of frames"() -> (w611:sgl)
              n1325 = local read "Y-lines"() -> (w612:sgl)
              n1326 = Multiply(x=w612, y=w611) -> (x*y=w610:sgl)
            }
          }
          n1327 = case shown="4" w575 {
            tunnel: w499 -> [_ w850 w882 w1054 w1235]
            tunnel: "Play Movie" -> [_ w849 w883 w1056 w1234]
            tunnel: "SlideHorizontal" -> [_ _ _ w1055 w1233]
            tunnel: w567 -> [_ _ w884 w1061 w1232]
            tunnel: w541 -> [_ _ w880 w1059 w1231]
            tunnel: [_ _ w886 w1058 w1230] -> w540
            tunnel: w539 -> [_ _ w881 w1060 w1229]
            tunnel: [_ _ w885 w1057 w1228] -> w538
            tunnel: w500 -> [_ _ w879 _ _]
            tunnel: w488 -> [w846 _ _ w1053 w1227]
            tunnel: w487 -> [w845 _ _ w1052 w1226]
            tunnel: w489 -> [w844 w848 w878 w1051 w1225]
            tunnel: w490 -> [w843 w847 w877 w1050 w1224]
            frame 0, Default {
              n1328 = local write "Image 2"(w843) -> ()
              n1329 = local write "Image 1"(w844) -> ()
              n1330 = local write "Image 3"(w846) -> ()
              n1331 = local write "Image 4"(w845) -> ()
            }
            frame 1 {
              n1332 = case shown="True" w849 {
                tunnel: w850 -> [_ w873]
                tunnel: w848 -> [w852 w869]
                tunnel: w847 -> [w851 w868]
                frame True {
                  n1333 = local read "Number of frames"() -> (w853:sgl)
                  n1334 = while {
                    shift-right: [w864] -> _
                    shift-left: i16 0 ("y") -> [w865]
                    tunnel: w853 -> [w863]
                    tunnel: w852 -> [w856]
                    tunnel: w851 -> [w855]
                    stop <- w861 stop-if-true
                    n1335 = local read "Y-lines"() -> (w858:sgl)
                    n1336 = call "ResetToZeroFOCUS.vi"("UpperLimit"=w863, "Running Index"=w865) -> ("New Index"=w860:i32)
                    n1337 = local read "Play Movie"() -> (w862:bool)
                    n1338 = Multiply(x=w860, y=w858) -> (x*y=w857:sgl)
                    n1339 = local write "ImageSlide"(w860) -> ()
                    n1340 = Not(x=w862) -> (.not. x?=w861:bool)
                    n1341 = Array Subset(array=w856, index (col)=w857, length (col)=w858) -> (w867:u8[][])  [unwired: 2 in]
                    n1342 = Array Subset(array=w855, index (col)=w857, length (col)=w858) -> (w866:u8[][])  [unwired: 2 in]
                    n1343 = Increment(x=w860) -> (x+1=w864:i32)
                    n1344 = local write "Image 2"(w866) -> ()
                    n1345 = local write "Image 1"(w867) -> ()
                    n1346 = Wait Until Next ms Multiple(millisecond multiple="Velocity") -> ()  [unwired: 1 out]
                  }
                }
                frame False {
                  n1347 = local read "Y-lines"() -> (w874:sgl)
                  n1348 = Round To Nearest(number=w873) -> (nearest integer value=w872:u32)
                  n1349 = Multiply(x=w874, y=w872) -> (x*y=w870:sgl)
                  n1350 = local read "Y-lines"() -> (w871:sgl)
                  n1351 = Array Subset(array=w869, index (col)=w870, length (col)=w871) -> (w876:u8[][])  [unwired: 2 in]
                  n1352 = Array Subset(array=w868, index (col)=w870, length (col)=w871) -> (w875:u8[][])  [unwired: 2 in]
                  n1353 = local write "Image 2"(w875) -> ()
                  n1354 = local write "Image 1"(w876) -> ()
                }
              }
            }
            frame 2 {
              n1355 = case shown="False" w883 {
                tunnel: w884 -> [w943 _]
                tunnel: [w938 _] -> w886
                tunnel: [w930 _] -> w885
                tunnel: w881 -> [w906 _]
                tunnel: w880 -> [w905 _]
                tunnel: w882 -> [w904 _]
                tunnel: w879 -> [w889 _]
                tunnel: w878 -> [w888 w1028]
                tunnel: w877 -> [w887 w1027]
                frame False {
                  w957 = 0.0
                  w941 = 0.0 ("Scale.Range:Minimum")
                  n1356 = local read "Reset1"() -> (w915:bool)
                  n1357 = local read "index (row)2"() -> (w901:i32)
                  n1358 = local read "Reset2"() -> (w916:bool)
                  n1359 = local read "index (row)1"() -> (w903:i32)
                  n1360 = local read "Y-lines"() -> (w893:sgl)
                  n1361 = local read "Average1"() -> (w902:i32)
                  n1362 = Subtract(x=w889, y=w902) -> (x-y=w942:sgl)
                  n1363 = local read "Number of frames"() -> (w894:sgl)
                  n1364 = local read "Average2"() -> (w900:i32)
                  n1365 = Subtract(x=w889, y=w900) -> (x-y=w940:sgl)
                  n1366 = local read "X-pixels"() -> (w958:sgl)
                  n1367 = Multiply(x=w893, y=w894) -> (x*y=w892:sgl)
